vi "update states from tdms.vi"(8 "error in (no error)":errorcluster, 10 "frot panel referances":T1, 11 "5785_2_x_200MHz in":refnum<class "5785_2_x_200MHz.lvclass">) -> (0 "error out":errorcluster, 2 "tdms file mode":T2=enum."P2P - VST", 3 "5785_2_x_200MHz out":refnum<class "5785_2_x_200MHz.lvclass">)   [LabVIEW 2021, in "5785_2_x_200MHz.lvclass"]
uses:
  5785_2_x_200MHz.lvclass
  5785_2_x_200MHz.lvclass/5785_2_x_200MHz.ctl
  pulse_tx_vis/device_mode.ctl
  device_type/device_type.lvclass
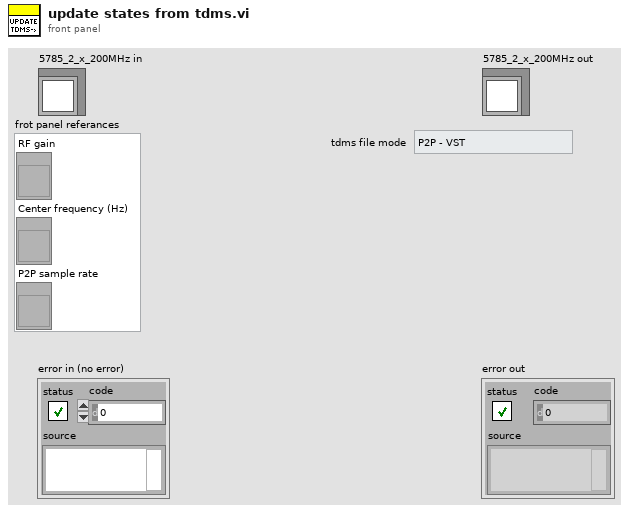
[diagram p1: front panel]
types:
  T1 = cluster{"RF gain ":refnum<vi>, "Center frequency (Hz) ":refnum<vi>, "P2P sample rate":refnum<vi>}
  T2 = typedef "device_mode.ctl" = enum16{"USRP - 180MHz", "5785 - 2*180MHz", "5785 - 3.2GHz", "P2P - VST"}
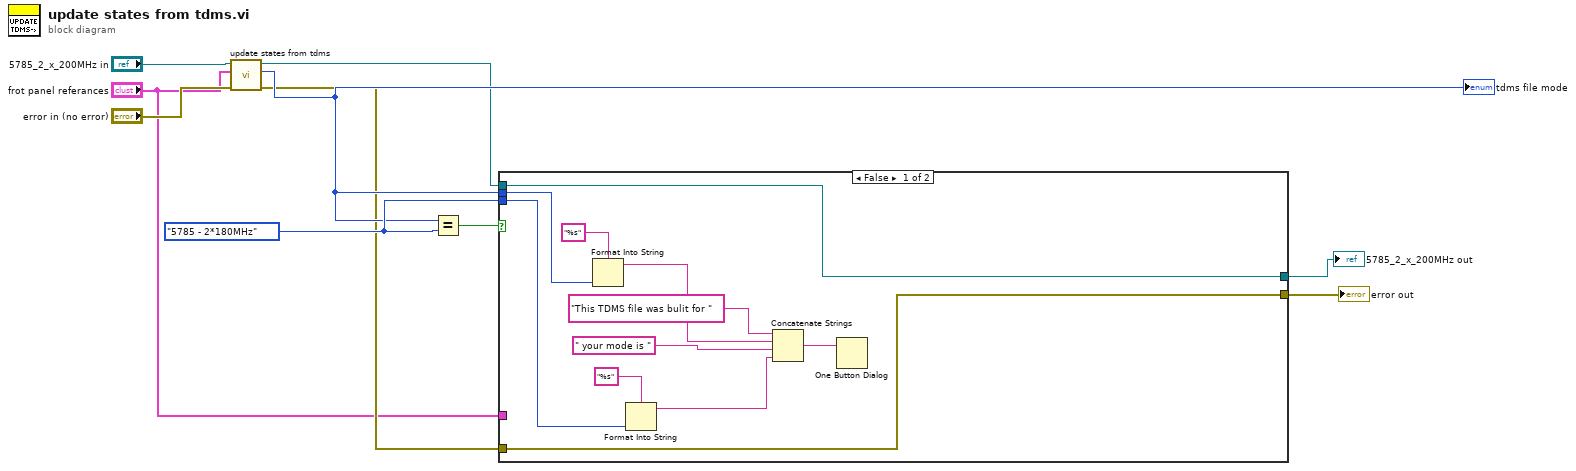
[diagram p0: block diagram]
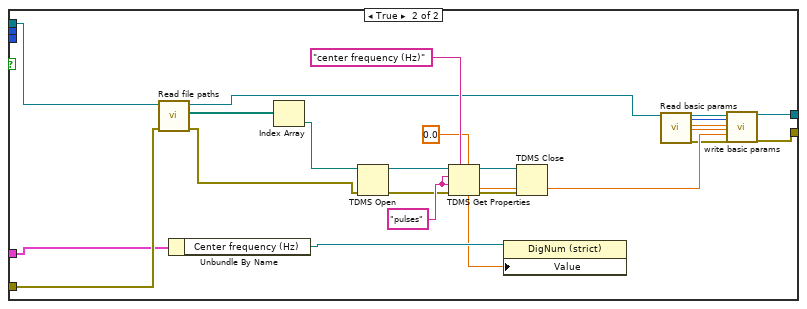
[diagram p2: hidden frame]
diagram:
  w7 = device_mode."5785 - 2*180MHz" ("Mode")
  n1 = call-parent "update states from tdms.vi"("error in (no error)"="error in (no error)", "frot panel referances"="frot panel referances", "device_type in"="5785_2_x_200MHz in") -> ("error out"=w5:errorcluster, "tdms file mode"=w6:T2, "device_type out"=w4:refnum<class "5785_2_x_200MHz.lvclass">)  [unwired: 6 in]
  "tdms file mode" <- w6
  n2 = Equal?(x=w6, y=w7) -> (x = y?=w8:bool)
  n3 = case shown="False" w8 {
    tunnel: w6 -> [w20 _]
    tunnel: w7 -> [w15 _]
    tunnel: w5 -> [w11 w37]
    tunnel: w4 -> [w12 w35]
    tunnel: "frot panel referances" -> [_ w32]
    tunnel: [w12 w23] -> w2
    tunnel: [w11 w22] -> w1
    frame False {
      n4 = Format Into String(format string="%s", w20) -> (resulting string=w19:string)  [unwired: 2 in, 1 out]
      n5 = Format Into String(format string="%s", w15) -> (resulting string=w14:string)  [unwired: 2 in, 1 out]
      n6 = Concatenate Strings("This TDMS file was bulit for " ("string"), w19, " your mode is " ("string"), w14) -> (w13:string)
      n7 = One Button Dialog(message=w13) -> ()  [unwired: 1 in, 1 out]
    }
    frame True {
      w44 = "pulses" ("channel name")
      n8 = call-dynamic "Read file paths.vi"("error in (no error)"=w37, "device_type in"=w35) -> ("error out"=w38:errorcluster, "file paths"=w36:path[], "device_type out"=w30:refnum<class "5785_2_x_200MHz.lvclass">)  [unwired: 7 in]
      n9 = Unbundle By Name(w32) -> ("Center frequency (Hz)"=w31:refnum<vi>)
      n10 = Index Array(array=w36) -> (element=w39:path)  [unwired: 1 in]
      n11 = TDMS Open(8:w38, 11:w39) -> (0:w42:errorcluster, 3:w43:refnum<k34>)  [unwired: 5 in]
      n12 = TDMS Get Properties(5:0.0, 7:"center frequency (Hz)", 8:w42, 9:w44, 10:w44, 11:w43) -> (0:w40:errorcluster, 3:w41:refnum<k34>, 4:w25:dbl)  [unwired: 3 out]
      n13 = property class="DigNum (strict)"(reference=w31, "Value"=w25) -> ()  [unwired: 1 in, 2 out]
      n14 = TDMS Close(8:w40, 11:w41) -> ()  [unwired: 2 out]
      n15 = call-dynamic "Read basic params.vi"("device_type in"=w30) -> ("device_type out"=w29:refnum<class "5785_2_x_200MHz.lvclass">, "buffer size"=w28:u32, "Fs  FPGA"=w27:dbl, "SPC"=w26:dbl, "error out"=w24:errorcluster)  [unwired: 13 in, 1 out]
      n16 = call-dynamic "write basic params.vi"("device_type in"=w29, "buffer size"=w28, "Fs  FPGA"=w27, "SPC"=w26, "center frequency (Hz)"=w25, "error in (no error)"=w24) -> ("device_type out"=w23:refnum<class "5785_2_x_200MHz.lvclass">, "error out"=w22:errorcluster)  [unwired: 12 in]
    }
  }
  "error out" <- w1
  "5785_2_x_200MHz out" <- w2
